vi "RSNRPZ Get Device Status Z5.vi"(8 "error in (no error)":errorcluster, 11 "VISA session":refnum<visa-resource-name> caption="VISA resource name") -> (0 "error out":errorcluster, 2 "Availability":i32, 3 "dup VISA session":refnum<visa-resource-name> caption="VISA resource name")   [LabVIEW 2010]
doc: "This VIs provides information about whether an NRP-Z5 is connected to the PC."
uses:
  rsnrpz_32.dll
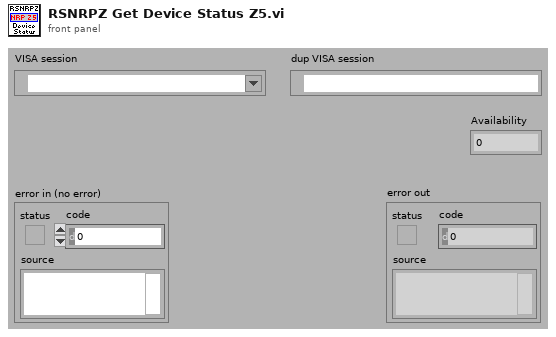
[diagram p1: front panel]
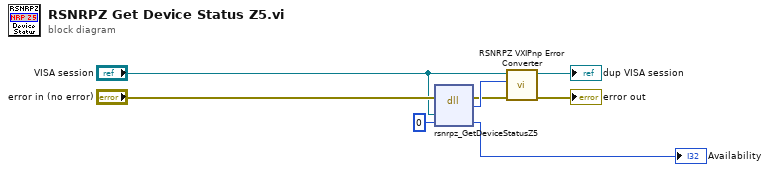
[diagram p0: block diagram]
diagram:
  n1 = dll-call lib="rsnrpz_32.dll" fn="rsnrpz_GetDeviceStatusZ5"(error in="error in (no error)", "Instrument Handle"="VISA session", "Availability"=0) -> (error out=w5:errorcluster, w7:i32, "Availability"=→"Availability":i32)  [unwired: 3 in, 1 out]
  n2 = call <instrlib>:"RSNRPZ VXIPnp Error Converter.vi"("error in"=w5, "VXIPnp error code"=w7, "VISA session"="VISA session") -> ("error out"=→"error out":errorcluster, "dup VISA session"=→"dup VISA session":refnum<visa-resource-name>)  [unwired: 7 in]
